vi "Comments.Create Lockin AO Description.vi"(7 "error in (no error)":errorcluster, 10 "Control Experiment":refnum<class "Control Experiment.lvclass">) -> (0 "error out":errorcluster, 2 "AO Section":string, 3 "Control Experiment out":refnum<class "Control Experiment.lvclass">)   [LabVIEW 2019, in "Control Experiment.lvclass"]
uses:
  <userlib>/LevyLab/Transport/Control Experiment/Control Experiment.lvclass
  <userlib>/LevyLab/Transport/Control Experiment/Control Experiment.lvclass/Control Experiment.ctl
  <userlib>/LevyLab/Lockin-Multichannel/Instrument.Lockin/Instrument.Lockin.lvclass
  <userlib>/LevyLab/PLYM/YAML.lvclass
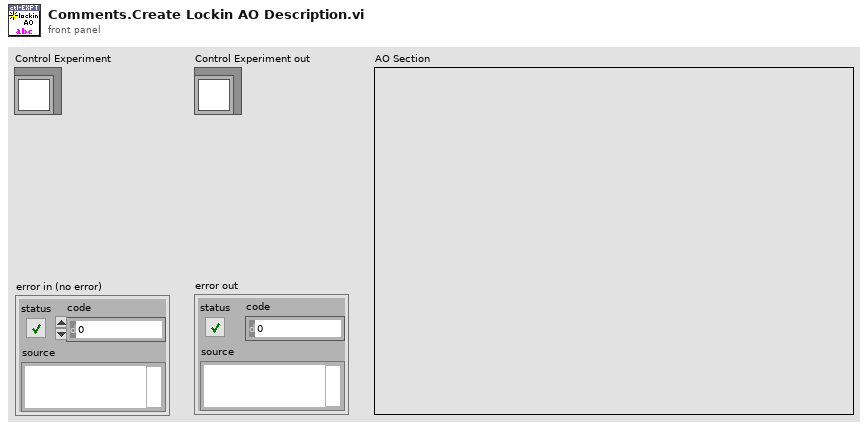
[diagram p1: front panel]
types:
  T1 = typedef "Instrument.DAQ.lvclass/AO.Channel--Cluster--Array.ctl" = T2[]
  T2 = typedef "Instrument.DAQ.lvclass/AO.Channel--Cluster.ctl" = cluster{"Enable?":bool, "Channel":i32, "Amplitude":dbl, "Offset":dbl, "Frequency":dbl, "Phase":dbl, "Function":T3, "Sweeping?":bool}
  T3 = typedef "Instrument.DAQ.lvclass/AO.Channel.Function--Enum.ctl" = enum16{"Sine", "Triangle", "Square"}
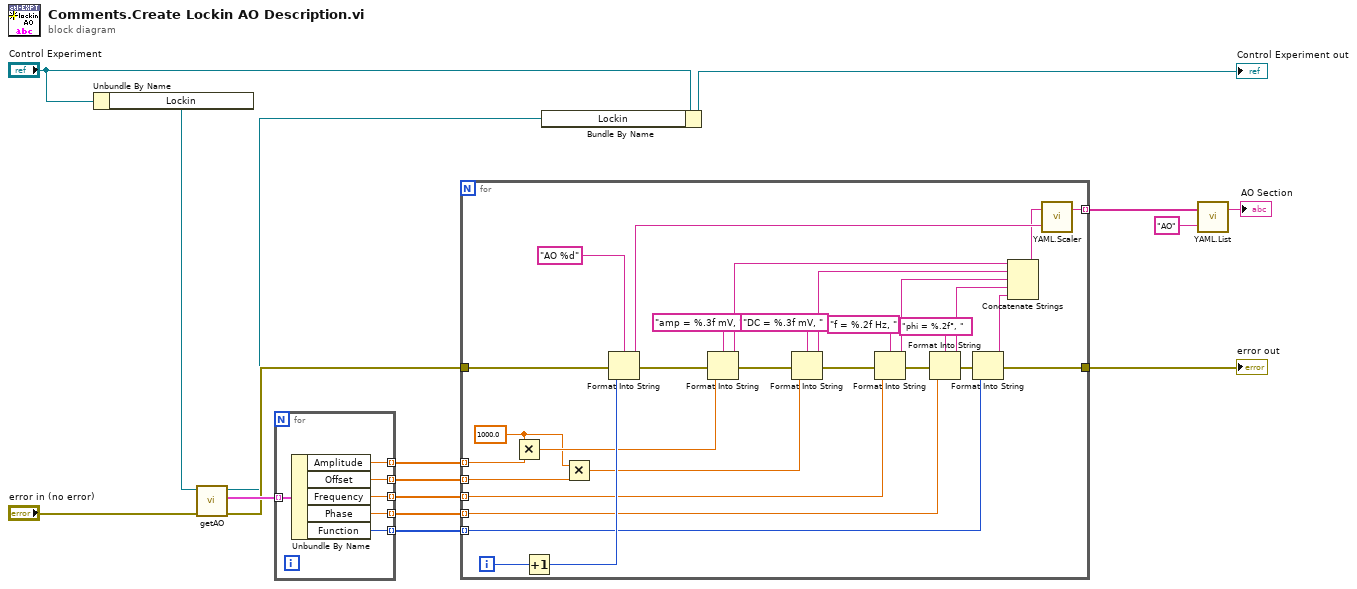
[diagram p0: block diagram]
diagram:
  n1 = Unbundle By Name("Control Experiment") -> ("Lockin"=w4:refnum<class "Instrument.Lockin.lvclass">)
  n2 = call <userlib>:"getAO.vi"("error in (no error)"="error in (no error)", "Instrument.Lockin in"=w4) -> ("error out"=w5:errorcluster, "AOconfig"=w6:T1, "Instrument.Lockin out"=w1:refnum<class "Instrument.Lockin.lvclass">)  [unwired: 7 in]
  n3 = for {
    tunnel: [w22] -> w12 mode=indexing
    tunnel: [w21] -> w11 mode=indexing
    tunnel: [w20] -> w10 mode=indexing
    tunnel: [w19] -> w9 mode=indexing
    tunnel: [w18] -> w8 mode=indexing
    tunnel: w6 -> [w17] mode=indexing
    n4 = Unbundle By Name(w17) -> ("Amplitude"=w22:dbl, "Offset"=w21:dbl, "Frequency"=w20:dbl, "Phase"=w19:dbl, "Function"=w18:T3)
  }
  n5 = for {
    tunnel: w12 -> [w29] mode=indexing
    tunnel: w11 -> [w30] mode=indexing
    tunnel: w10 -> [w37] mode=indexing
    tunnel: w9 -> [w35] mode=indexing
    tunnel: w8 -> [w36] mode=indexing
    tunnel: [w23] -> w7 mode=indexing
    tunnel: w5 -> [w52]
    tunnel: [w47] -> w16
    i -> [w45]
    w26 = 1000.0 ("x")
    n6 = Multiply(x=w26, y=w29) -> (x*y=w27:dbl)
    n7 = Increment(x=w45) -> (x+1=w40:i32)
    n8 = Multiply(x=w26, y=w30) -> (x*y=w28:dbl)
    n9 = Format Into String(format string="AO %d", error in=w52, w40) -> (resulting string=w25:string, error out=w51:errorcluster)  [unwired: 1 in]
    n10 = Format Into String(format string="amp = %.3f mV, ", error in=w51, w27) -> (resulting string=w42:string, error out=w46:errorcluster)  [unwired: 1 in]
    n11 = Format Into String(format string="DC = %.3f mV, ", error in=w46, w28) -> (resulting string=w39:string, error out=w50:errorcluster)  [unwired: 1 in]
    n12 = Format Into String(format string="f = %.2f Hz, ", error in=w50, w37) -> (resulting string=w34:string, error out=w49:errorcluster)  [unwired: 1 in]
    n13 = Format Into String(format string="phi = %.2f°, ", error in=w49, w35) -> (resulting string=w32:string, error out=w48:errorcluster)  [unwired: 1 in]
    n14 = Format Into String(error in=w48, w36) -> (resulting string=w31:string, error out=w47:errorcluster)  [unwired: 2 in]
    n15 = Concatenate Strings(w42, w39, w34, w32, w31) -> (w24:string)
    n16 = call <userlib>:"YAML.Scaler.vi"("Key"=w25, "Scaler"=w24) -> ("Output"=w23:string)  [unwired: 1 in]
  }
  "error out" <- w16
  n17 = Bundle By Name(cluster="Control Experiment", "Lockin"=w1) -> (→"Control Experiment out":refnum<class "Control Experiment.lvclass">)
  n18 = call <userlib>:"YAML.List.vi"("Key"="AO" ("string"), "lines"=w7) -> ("Output"=→"AO Section":string)  [unwired: 1 in]
